vi "TestDAQAOInit.vi"(4 "ConfigData":string, 5 "DAQName":string) -> (0 "Parameter OK":bool, 1 "DAQData":T1, 2 "VI Refnum":refnum<vi>)   [LabVIEW 2020]
uses:
  <vilib>/DAQmx/create/channels.llb/DAQmx Create Channel (AO-Voltage-Basic).vi
panel:
  out "IO":string
  out "InitOK?":bool
  in  "DAQTask":refnum<k21>
  in  "SPS":dbl
  in  "Len":dbl
  in  "Min":dbl
  in  "Max":dbl
  in  "CH":string
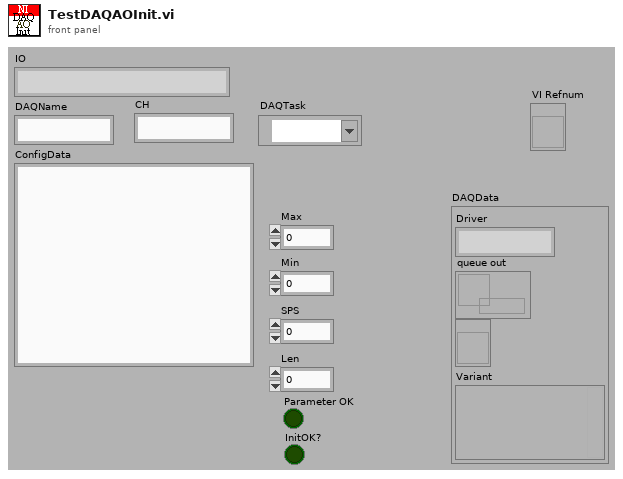
[diagram p1: front panel]
types:
  T1 = cluster{"Driver":string, "queue out":refnum<queue>, refnum<vi>, "Variant":variant}
  T2 = cluster{"Command":string, "Parameter":string, "queue out":refnum<queue>}
  T3 = cluster{"DAQTask":refnum<k21>, "DAQName":string, "CH":string, "Max":dbl, "Min":dbl, "SPS":dbl, "Len":dbl}
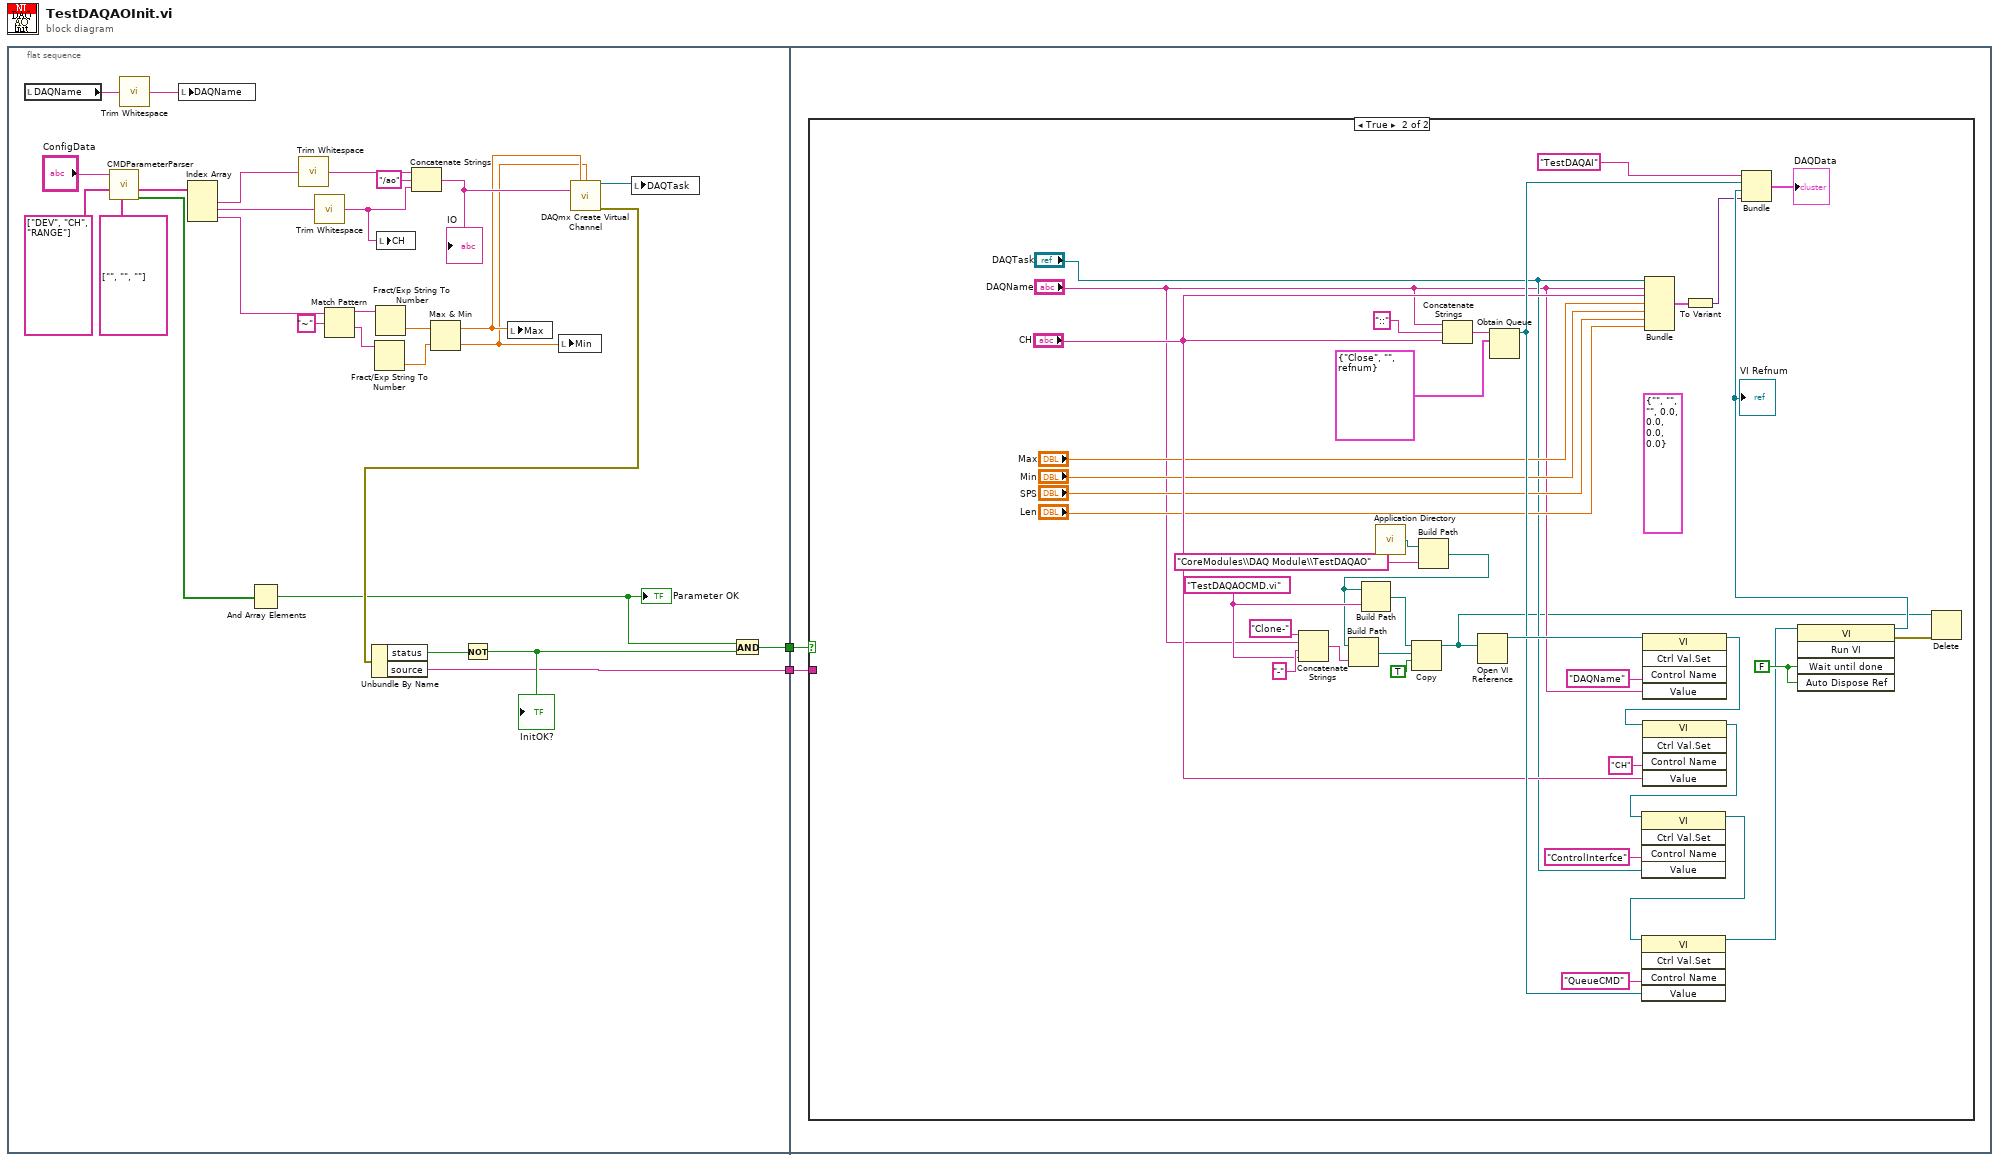
[diagram p0: block diagram]
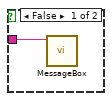
[diagram p2: hidden frame]
diagram:
  n1 = flat-sequence {
    tunnel: [w22] -> w2
    tunnel: [w12] -> w1
    tunnel: w2 -> [w32]
    tunnel: w1 -> [w31]
    frame #0 {
      n2 = local read "DAQName"() -> (w23:string)
      n3 = call "CMDParameterParser.vi"("DeafultValues"=string[] ["", "", ""] ("ParameterKey"), "RequiredKeys"=string[] ["DEV", "CH", "RANGE"] ("ParameterKey"), "CMDParameter"="ConfigData") -> ("KeyFind?"=w4:bool[], "KeyValues"=w8:string[])  [unwired: 6 in, 1 out]
      n4 = call <vilib>:"Trim Whitespace.vi"("string"=w23) -> ("trimmed string"=w24:string)  [unwired: 1 in]
      n5 = local write "DAQName"(w24) -> ()
      n6 = Index Array(array=w8) -> (element #1=w7:string, element #2=w6:string, element #3=w5:string)  [unwired: 3 in]
      n7 = And Array Elements(Boolean array=w4) -> (logical AND=w3:bool)
      "Parameter OK" <- w3
      n8 = call <vilib>:"Trim Whitespace.vi"("string"=w7) -> ("trimmed string"=w27:string)  [unwired: 1 in]
      n9 = call <vilib>:"Trim Whitespace.vi"("string"=w6) -> ("trimmed string"=w25:string)  [unwired: 1 in]
      n10 = Match Pattern(string=w5, regular expression="~") -> (before substring=w29:string, after substring=w28:string)  [unwired: 1 in, 2 out]
      n11 = Fract/Exp String To Number(string=w28) -> (number=w18:dbl)  [unwired: 3 in, 1 out]
      n12 = Fract/Exp String To Number(string=w29) -> (number=w19:dbl)  [unwired: 3 in, 1 out]
      n13 = local write "CH"(w25) -> ()
      n14 = Concatenate Strings(w27, "/ao" ("string"), w25) -> (w20:string)
      "IO" <- w20
      n15 = Max & Min(x=w19, y=w18) -> (max(x,y)=w17:dbl, min(x,y)=w16:dbl)
      n16 = local write "Max"(w17) -> ()
      n17 = local write "Min"(w16) -> ()
      n18 = call-poly <vilib>:"DAQmx Create Virtual Channel.vi"("maximum value"=w17, "minimum value"=w16, "physical channels"=w20) -> ("task out"=w15:refnum<k21>, "error out"=w14:errorcluster)  [unwired: 11 in]
      n19 = Unbundle By Name(w14) -> ("status"=w13:bool, "source"=w12:string)
      n20 = Not(x=w13) -> (.not. x?=w21:bool)
      "InitOK?" <- w21
      n21 = local write "DAQTask"(w15) -> ()
      n22 = And(x=w3, y=w21) -> (x .and. y?=w22:bool)
    }
    frame #1 {
      n23 = case shown="True" w32 {
        tunnel: w31 -> [w33 _]
        frame False {
          n24 = call "MessageBox.vi"("!!!!!!!!!!!!!Message!!!!!!!!!!!!!"=w33) -> ()  [unwired: 10 in, 1 out]
        }
        frame True {
          (unwired) T3 {"DAQTask"="", "DAQName"="", "CH"="", "Max"=0.0, "Min"=0.0, "SPS"=0.0, "Len"=0.0} ("output cluster")
          w51 = FALSE ("Wait Until Done")
          w62 = "TestDAQAOCMD.vi" ("name or relative path")
          n25 = Concatenate Strings("Clone-" ("string"), "DAQName", "-" ("string"), w62) -> (w66:string)
          n26 = call <vilib>:"Application Directory.vi"() -> ("Application Directory"=w45:path)
          n27 = Build Path(base path=w45, name or relative path="CoreModules\\DAQ Module\\TestDAQAO") -> (appended path=w44:path)
          n28 = Build Path(base path=w44, name or relative path=w66) -> (appended path=w64:path)
          n29 = Build Path(base path=w44, name or relative path=w62) -> (appended path=w61:path)
          n30 = Copy(9:TRUE ("overwrite (F)"), 10:w64, 11:w61) -> (3:w35:path)  [unwired: 2 in, 2 out]
          n31 = Concatenate Strings("DAQName", "::" ("string"), "CH") -> (w70:string)
          n32 = Open VI Reference(vi path=w35) -> (vi reference=w56:refnum<vi>)  [unwired: 5 in, 1 out]
          n33 = Obtain Queue(name (unnamed)=w70, element data type=T2 {"Command"="Close", "Parameter"="", "queue out"=refnum} ("Motor Module CMD")) -> (queue out=w55:refnum<queue>)  [unwired: 3 in, 2 out]
          n34 = invoke class="VI" method="Ctrl Val.Set"(reference=w56, "Control Name"="DAQName", "Value"="DAQName") -> (reference out=w54:refnum<vi>)  [unwired: 2 in, 4 out]
          n35 = invoke class="VI" method="Ctrl Val.Set"(reference=w54, "Control Name"="CH", "Value"="CH") -> (reference out=w53:refnum<vi>)  [unwired: 2 in, 4 out]
          n36 = invoke class="VI" method="Ctrl Val.Set"(reference=w53, "Control Name"="ControlInterfce", "Value"="DAQTask") -> (reference out=w52:refnum<vi>)  [unwired: 2 in, 4 out]
          n37 = invoke class="VI" method="Ctrl Val.Set"(reference=w52, "Control Name"="QueueCMD", "Value"=w55) -> (reference out=w34:refnum<vi>)  [unwired: 2 in, 4 out]
          n38 = Bundle("DAQTask"="DAQTask", "DAQName"="DAQName", "CH"="CH", "Max"="Max", "Min"="Min", "SPS"="SPS", "Len"="Len") -> (w71:T3)  [unwired: 1 in]
          n39 = To Variant(anything=w71) -> (Variant=w48:variant)
          n40 = invoke class="VI" method="Run VI"(reference=w34, "Wait until done"=w51, "Auto Dispose Ref"=w51) -> (reference out=w49:refnum<vi>, error out=w36:errorcluster)  [unwired: 2 in, 3 out]
          "VI Refnum" <- w49
          n41 = Bundle("Driver"="TestDAQAI", "queue out"=w55, w49, "Variant"=w48) -> (→"DAQData":T1)  [unwired: 1 in]
          n42 = Delete(path (use dialog)=w35, error in=w36) -> ()  [unwired: 3 in, 3 out]
        }
      }
    }
  }
